vi "Raw Text to 1D String.vi"(8 "Error In":errorcluster, 9 "Use Example Input":bool, 10 "Example Input":string, 11 "Relative Path to Input File":string) -> (0 "Error Out":errorcluster, 3 "1D String Array":string[](array[string]))   [LabVIEW 2019]
doc: "Given a relative path, retrieve a 1D string array from an input text file. This assumes Line Feed delimiters."
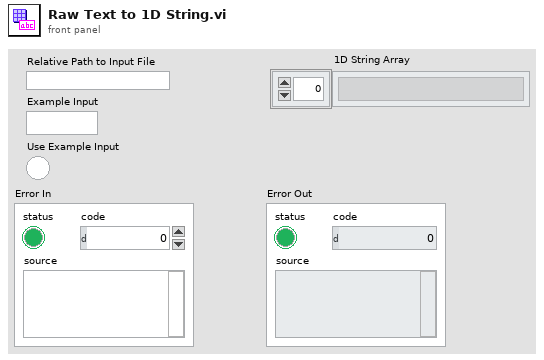
[diagram p1: front panel]
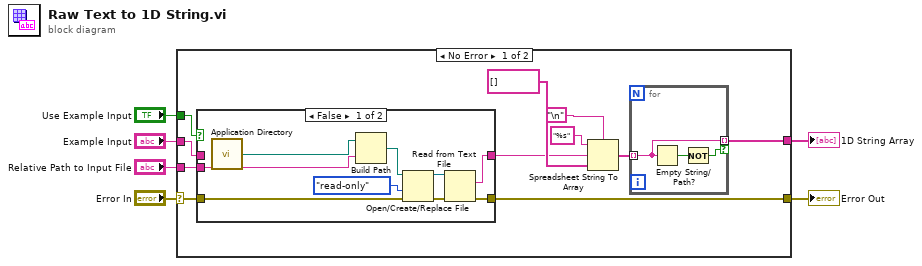
[diagram p0: block diagram]
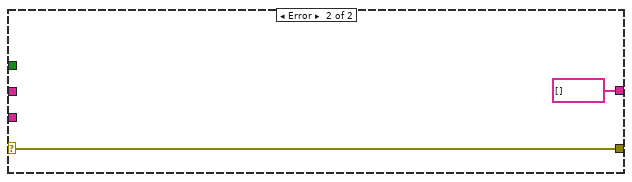
[diagram p3: hidden frame]
diagram:
  n1 = case shown="No Error" "Error In" {
    selector: "Error In" -> [w11 w33]
    tunnel: "Relative Path to Input File" -> [w17 _]
    tunnel: [w7 string[] []] -> w5
    tunnel: [w13 w33] -> w4
    tunnel: "Use Example Input" -> [w10 _]
    tunnel: "Example Input" -> [w9 _]
    frame No Error {
      n2 = case shown="False" w10 {
        tunnel: w17 -> [w28 _]
        tunnel: [w23 w31] -> w15
        tunnel: [w22 w30] -> w13
        tunnel: w11 -> [w21 w30]
        tunnel: w9 -> [_ w31]
        frame False {
          n3 = call <vilib>:"Application Directory.vi"() -> ("Application Directory"=w29:path)
          n4 = Build Path(base path=w29, name or relative path=w28) -> (appended path=w27:path)
          n5 = Open/Create/Replace File(file path (use dialog)=w27, error in=w21, access (0:read/write)=enum16{"read/write", "read-only", "write-only"}."read-only") -> (refnum out=w25:refnum<file>, error out=w24:errorcluster)  [unwired: 3 in, 1 out]
          n6 = Read from Text File(file (use dialog)=w25, error in=w24) -> (text=w23:string, error out=w22:errorcluster)  [unwired: 2 in, 2 out]
        }
        frame True {
        }
      }
      n7 = Spreadsheet String To Array(delimiter (Tab)="\n", format string="%s", spreadsheet string=w15, array type (2D Dbl)=string[] []) -> (array=w8:string[])
      n8 = for {
        tunnel: w8 -> [w20] mode=indexing
        tunnel: [w20] -> w7 mode=indexing if=w18
        n9 = Empty String/Path?(string/path=w20) -> (empty?=w19:bool)
        n10 = Not(x=w19) -> (.not. x?=w18:bool)
      }
    }
    frame Error {
    }
  }
  "Error Out" <- w4
  "1D String Array" <- w5
